vi "SimpleProject.vi"() -> ()   [LabVIEW 2019]
panel:
  in  "Boolean":bool
  out "Temprature  vary chart":dbl[](graph)
  out "Temprature  of slide":dbl
  in  "Slide":dbl(slide) scale=0.0..10.0
  out "size of Thermometre array":i32
  out "Vertical slider thermometre":dbl[](array[slide]) scale=0.0..10.0
  out "String 2":string
  in  "Array":string[](array[string])
  out "Numeric 2":dbl
  in  "Numeric":dbl
  out "String":string
  # "On"
  # "Off"
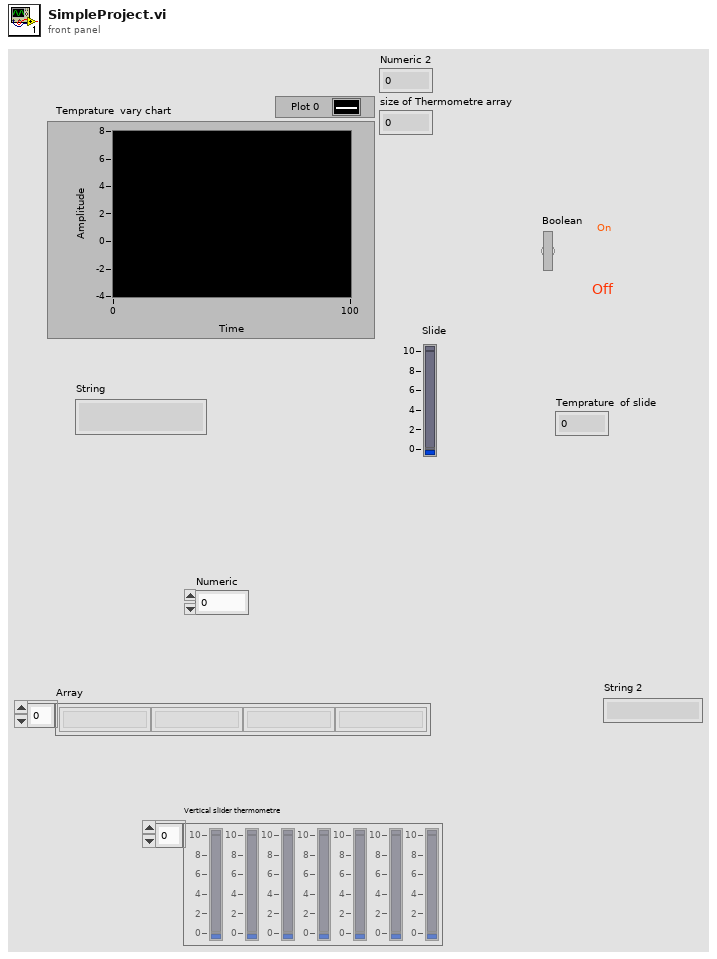
[diagram p1: front panel]
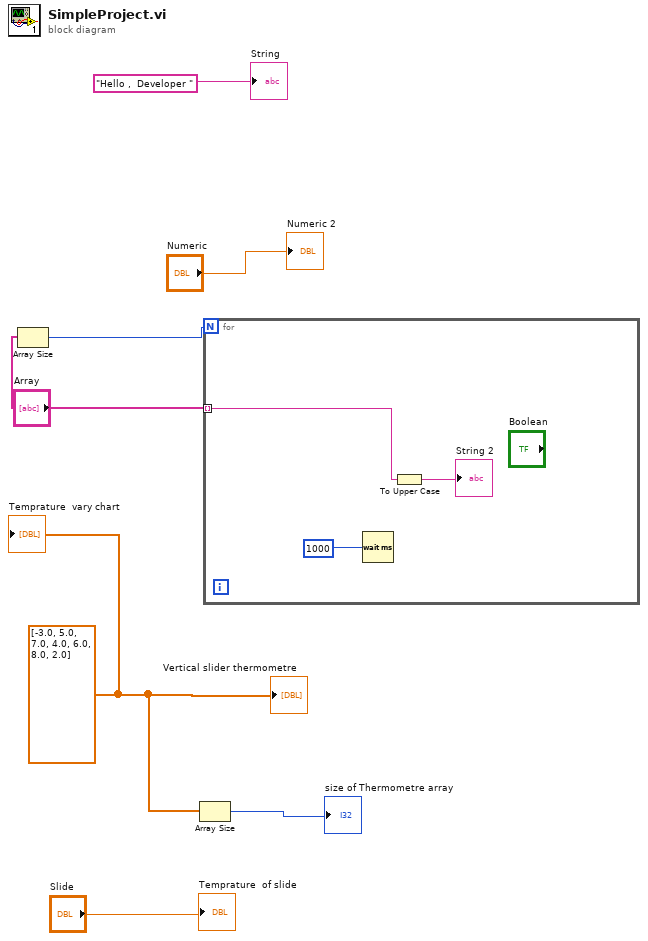
[diagram p0: block diagram]
diagram:
  w1 = dbl[] [-3.0, 5.0, 7.0, 4.0, 6.0, 8.0, 2.0] ("Vertical slider thermometre")
  n1 = Array Size(array="Array") -> (size(s)=w5:i32)
  n2 = Array Size(array=w1) -> (size(s)=→"size of Thermometre array":i32)
  n3 = for {
    N: w5 -> [_]
    tunnel: "Array" -> [w8] mode=indexing
    n4 = Wait (ms)(milliseconds to wait=u32 1000) -> ()  [unwired: 1 out]
    n5 = To Upper Case(1:w8) -> (0:→"String 2":string)
  }
  "String" <- "Hello ,  Developer " ("String")
  "Numeric 2" <- "Numeric"
  "Vertical slider thermometre" <- w1
  "Temprature  of slide" <- "Slide"
  "Temprature  vary chart" <- w1
